vi "Get File From Redis.vi"() -> ()   [LabVIEW 2019, in "HTTP Server.lvlib"]
uses:
  HTTP Server.lvlib
  REDIS/Palette/Redis Commands/Connection/AUTH.vi
  REDIS/Palette/Redis Commands/Connection/SELECT.vi
  REDIS/Palette/Redis Commands/Hashes/HGET.vi
panel:
  in  "文件路径（使用对话框）":path
  out "error out":errorcluster
  out "error out 2":errorcluster
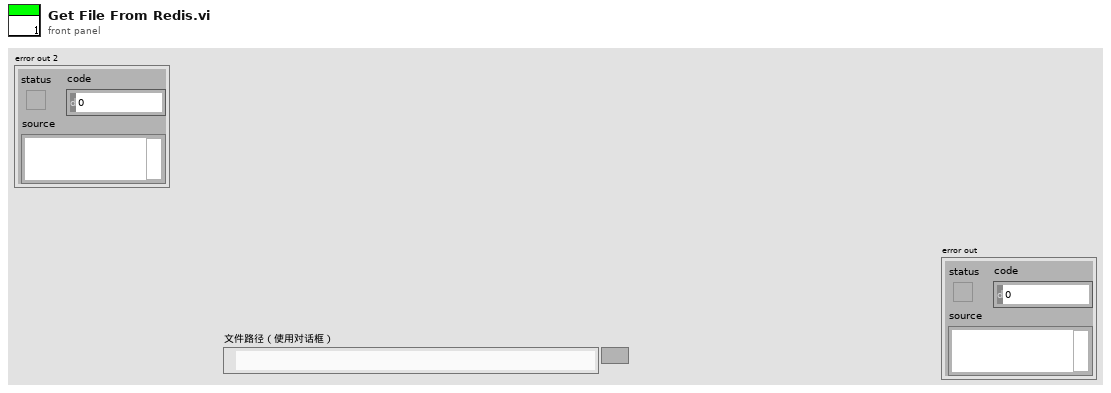
[diagram p1: front panel]
types:
  T1 = enum16{"open", "replace", "create", "open or create", "replace or create", "replace or create with confirmation"}
  T2 = typedef "redis-data.ctl" = cluster{"type":enum16{"None", "Error", "Status", "Nil", "Integer", "String", "Multibulk"}, "integer":i64, "string":string, "multibulk":variant[], "string data":string[]}
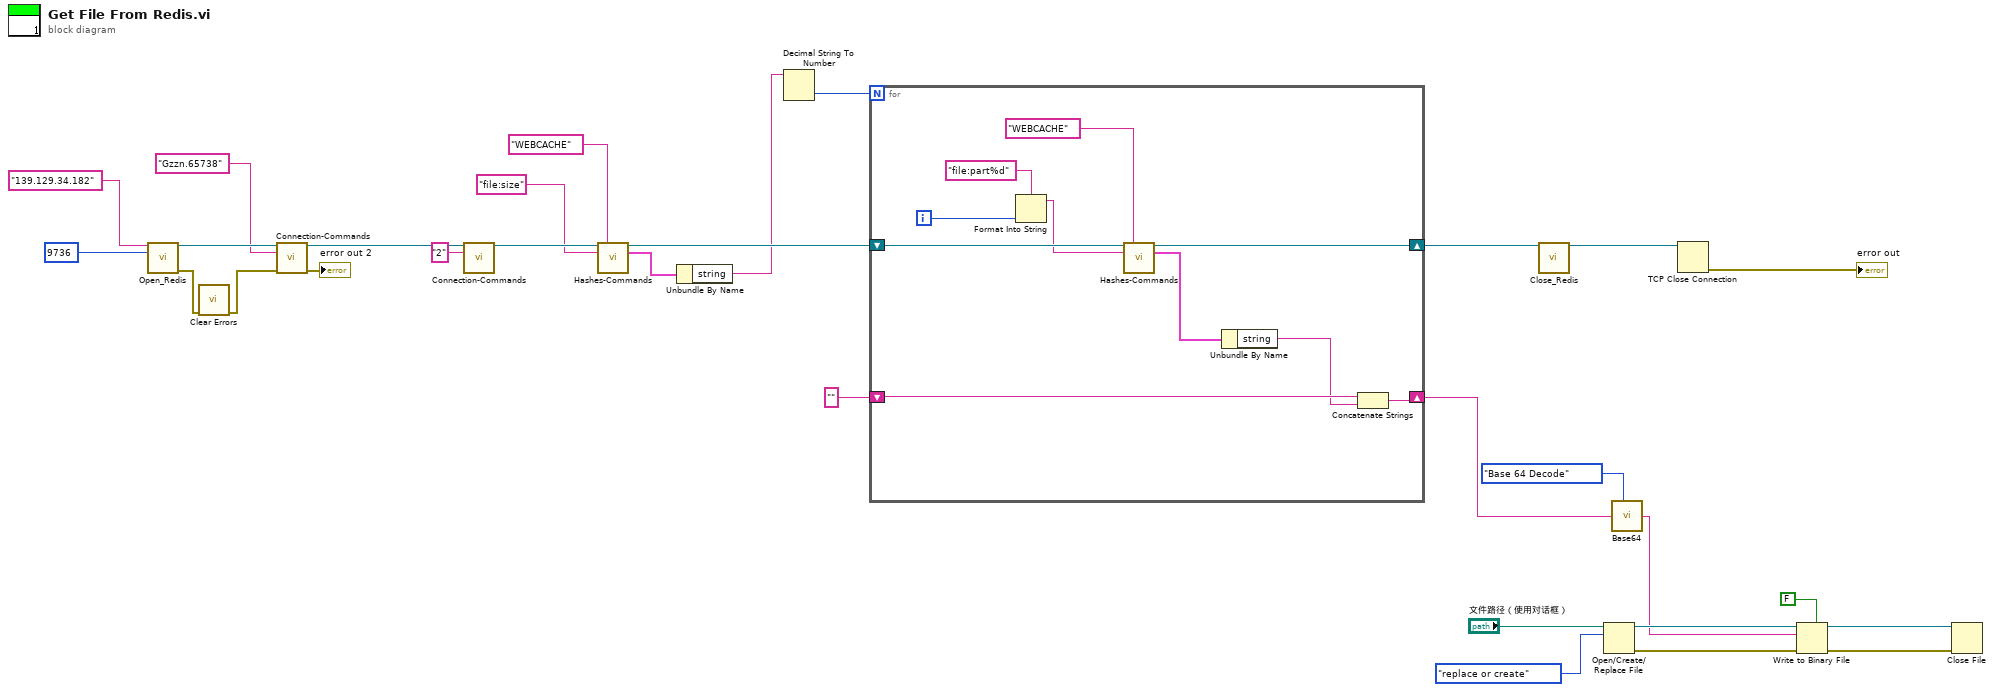
[diagram p0: block diagram]
diagram:
  n1 = call "Open_Redis.vi"("Host"="139.129.34.182", "Port"=u16 9736) -> ("redis连接ID"=w28:refnum<k5>, "error out"=w24:errorcluster)  [unwired: 11 in, 1 out]
  n2 = call <vilib>:"Clear Errors.vi"("error in (no error)"=w24) -> ("error out"=w23:errorcluster)  [unwired: 5 in, 1 out]
  n3 = call-poly "Connection-Commands.vi"("redis连接ID"=w28, "字符串"="Gzzn.65738", "error in"=w23) -> ("redis连接ID"=w26:refnum<k5>, "error out"=→"error out 2":errorcluster)  [unwired: 10 in, 1 out]
  n4 = call-poly "Connection-Commands.vi"("redis连接ID"=w26, "index"="2") -> ("redis连接ID"=w16:refnum<k5>)  [unwired: 11 in, 2 out]
  n5 = call-poly "Hashes-Commands.vi"("redis连接ID"=w16, "Key"="WEBCACHE", "Field"="file:size") -> ("redis连接ID"=w15:refnum<k5>, "Data"=w12:T2)  [unwired: 10 in, 1 out]
  n6 = Unbundle By Name(w12) -> ("string"=w2:string)
  n7 = Decimal String To Number(string=w2) -> (number=w1:i32)  [unwired: 2 in, 1 out]
  n8 = for {
    N: w1 -> [_]
    shift-right: [w35] -> w19
    shift-left: w15 -> [w40]
    shift-right: [w31] -> w17
    shift-left: "" -> [w33]
    i -> [w37]
    n9 = Format Into String(format string="file:part%d" ("Key"), w37) -> (resulting string=w36:string)  [unwired: 2 in, 1 out]
    n10 = call-poly "Hashes-Commands.vi"("redis连接ID"=w40, "Key"="WEBCACHE", "Field"=w36) -> ("redis连接ID"=w35:refnum<k5>, "Data"=w34:T2)  [unwired: 10 in, 1 out]
    n11 = Unbundle By Name(w34) -> ("string"=w32:string)
    n12 = Concatenate Strings(w33, w32) -> (w31:string)
  }
  n13 = call "Close_Redis.vi"("redis连接ID"=w19) -> ("redis连接ID 2"=w21:refnum<k5>)  [unwired: 11 in, 3 out]
  n14 = Open/Create/Replace File(file path (use dialog)="文件路径（使用对话框）", operation (0:open)=T1."replace or create" ("操作(0:open)")) -> (refnum out=w10:refnum<file>, error out=w9:errorcluster)  [unwired: 4 in, 1 out]
  n15 = call "Base64.vi"("Switch"=enum16{"Base 64 Encode", "Base 64 Decode"}."Base 64 Decode", "Input String"=w17) -> ("Output String"=w5:string)  [unwired: 5 in]
  n16 = TCP Close Connection(connection ID=w21) -> (error out=→"error out":errorcluster)  [unwired: 2 in, 1 out]
  n17 = Write to Binary File(file (use dialog)=w10, data=w5, error in=w9, 5:FALSE ("预置数组或字符串大小？ (T)")) -> (refnum out=w8:refnum<file>, error out=w7:errorcluster)  [unwired: 2 in, 1 out]
  n18 = Close File(refnum=w8, error in=w7) -> ()  [unwired: 2 out]
